vi "Arm State Machine.vi"   [LabVIEW 2015]
uses:
  ArmStates.ctl
  <vilib>/Rock Robotics/WPI/DriverStation/WPI_DriverStationRobotMode2.ctl
  Robot Global Data.vi
  <vilib>/Rock Robotics/WPI/Utilities/WPI_GetSetVariantRefNum.vi
types:
  T1 = typedef "ArmStates.ctl" = enum16{"Arm Drive Position", "Winch Up", "Level Arm", "Hold Climb", "Drawbridge Drive Forward", "Shoot Position", "Roll Out", "Hic Up Rollers Off", "Draw Bridge Arm Down", "Harvest Back Down", "Harvest Hic up", "Portcullis", "Sally Door", "Harvest", "Arm Up", "Arm Down"}
  T2 = cluster{"Arm State":T1, "Current Arm Position":dbl, "Arm Base Offset":dbl, "Arm Up Position":dbl, "Sally Door Position":dbl, "Porticullis Position":dbl, "Drawbridge Position":dbl, "Drive Position":dbl, "Arm Hic Up Position":dbl, "Desired Arm Position":dbl, "Arm Power Vbus":bool, "Roller":bool, "Hic Up Counter":i32, "Right Drive Overide Speed":dbl, "Left Drive Overide Speed":dbl, "Overide Drives":bool, "Roller Speed":dbl, "PTO on":bool, "PTO break Off":bool, "Current Encoder Position":dbl, "Starting Encoder Position":dbl, "Last State":T1, "Arm Hold Cylinder":bool, "New Base Offset":bool}
  T3 = typedef "WPI_MotorControlDeviceRef.ctl" = cluster{"DeviceStatus":errorcluster, "Type":T4, "PWM":cluster{"PWM Channel":T5, "DeadBand":T6}, "CAN":cluster{"Device Number":u8, "Control Mode":T7, "Semaphore":T8, "Max Vout":dbl, "TalonSRX Control Mode":T9}, "Invert":bool}
  T4 = typedef "WPI_MotorControlType.ctl" = enum16{"PWM", "CAN", "CANTalonSRX"}
  T5 = typedef "FPGA_DIOPWMChannel.ctl" = enum8{"PWM 0", "PWM 1", "PWM 2", "PWM 3", "PWM 4", "PWM 5", "PWM 6", "PWM 7", "PWM 8", "PWM 9", "PWM MXP 0", "PWM MXP 1", "PWM MXP 2", "PWM MXP 3", "PWM MXP 4", "PWM MXP 5", "PWM MXP 6", "PWM MXP 7", "PWM MXP 8", "PWM MXP 9", "Invalid"}
  T6 = typedef "WPI_PWMDeadband.ctl" = cluster{"Name":string, "maxPositivePwm":i32, "minPositivePwm":i32, "centerPwm":i32, "maxNegativePwm":i32, "minNegativePwm":i32, "angularRange":u16}
  T7 = typedef "WPI_CANJaguar_ControlMode.ctl" = enum8{"Percent VBus", "Current", "Speed", "Position", "Voltage"}
  T8 = typedef "Semaphore RefNum" = refnum<k1>
  T9 = typedef "WPI_CANTalonSRX_APIControlMode.ctl" = enum8{"Percent VBus", "Speed", "Position", "Slave", "Unchanged / Invalid", "Voltage Compensation", "Current", "Motion Profile"}
  T10 = typedef "WPI_CANTalonSRX_GlobalStatus.ctl" = cluster{"Applied Throttle":dbl, "Module Enabled":bool, "CAN Error":errorcluster, "Closed Loop Error":dbl, "Forward Limit Switch Closed":bool, "Reverse Limit Switch Closed":bool, "Sensor Position":dbl, "Sensor Velocity":dbl, "Current":dbl, "Sticky Fault - Over Temp":bool, "Sticky Fault - Under Voltage":bool, "Sticky Fault - Forward Limit":bool, "Sticky Fault - Reverse Limit":bool, "Sticky Fault - Forward Soft Limit":bool, "Sticky Fault - Reverse Soft Limit":bool, "Brake is Enabled":bool, "Encoder Position":dbl, "Encoder Velocity":dbl, "Encoder Index Count":dbl, "Encoder A Pin State":bool, "Encoder B Pin State":bool, "Encoder Index Pin State":bool, "Analog In":dbl, "Analog In Velocity":dbl, "Temperature (C)":dbl, "Battery Voltage":dbl, "Control 5 Is Supported":bool, "Current Profile Slot Select":dbl, "Pos Div 8":bool, "Vel Div 4":bool, "Pulse Width Position":i32, "Pulse Width Velocity":i32, "Pulse Width Rise To Rise (us)":i32, "Pulse Width Rise To Fall (us)":i32, "Mot Prof Active Is Under Run":bool, "Mot Prof Active Has Under Run":bool, "Mot Prof Active Is Last":bool, "Mot Prof Active Velocity Only":bool, "Mot Prof Active Is Valid":bool, "Mot Prof Buffer Is Full":bool, "Mot Prof Active Profile Slot Select":i32, "Mot Prof NextID":i32, "Mot Prof Count":i32, "Mot Prof Active Velocity":dbl, "Mot Prof Active Position":dbl, "Mot Prof Output Enable":i32}
  T11 = typedef "WPI_DriverStationRobotMode2.ctl" = enum16{"Autonomous Disabled", "Autonomous Enabled", "Teleop Disabled", "Teleop Enabled", "Disconnected", "Finish", "Test Disabled", "Test Enabled", "Emergency Stopped"}
  T12 = typedef "WPI_JoystickDevRef.ctl" = cluster{"Device":T13}
  T13 = typedef "WPI_JoystickDeviceEnum.ctl" = enum16{"USB 0", "USB 1", "USB 2", "USB 3", "USB 4", "USB 5"}
  T14 = cluster{"Buttons[0]":bool, "Buttons[1]":bool, "Buttons[2]":bool, "Buttons[3]":bool, "Buttons[4]":bool, "Buttons[5]":bool, "Buttons[6]":bool, "Buttons[7]":bool, "Buttons[8]":bool}
  T15 = typedef "WPI_SwitchDevRef.ctl" = cluster{"DevStatus":errorcluster, "DIO Channel":T16, "CntIndex":T17, "Normally Closed":bool}
  T16 = typedef "FPGA_DIOChannel.ctl" = enum8{"DIO 0", "DIO 1", "DIO 2", "DIO 3", "DIO 4", "DIO 5", "DIO 6", "DIO 7", "DIO 8", "DIO 9", "DIO MXP 0", "DIO MXP 1", "DIO MXP 2", "DIO MXP 3", "DIO MXP 4", "DIO MXP 5", "DIO MXP 6", "DIO MXP 7", "DIO MXP 8", "DIO MXP 9", "DIO MXP 10", "DIO MXP 11", "DIO MXP 12", "DIO MXP 13", "DIO MXP 14", "DIO MXP 15", "Invalid"}
  T17 = typedef "FPGA_CounterCtrSystemIndex.ctl" = enum8{"Ctr 0", "Ctr 1", "Ctr 2", "Ctr 3", "Ctr 4", "Ctr 5", "Ctr 6", "Ctr 7", "Invalid"}
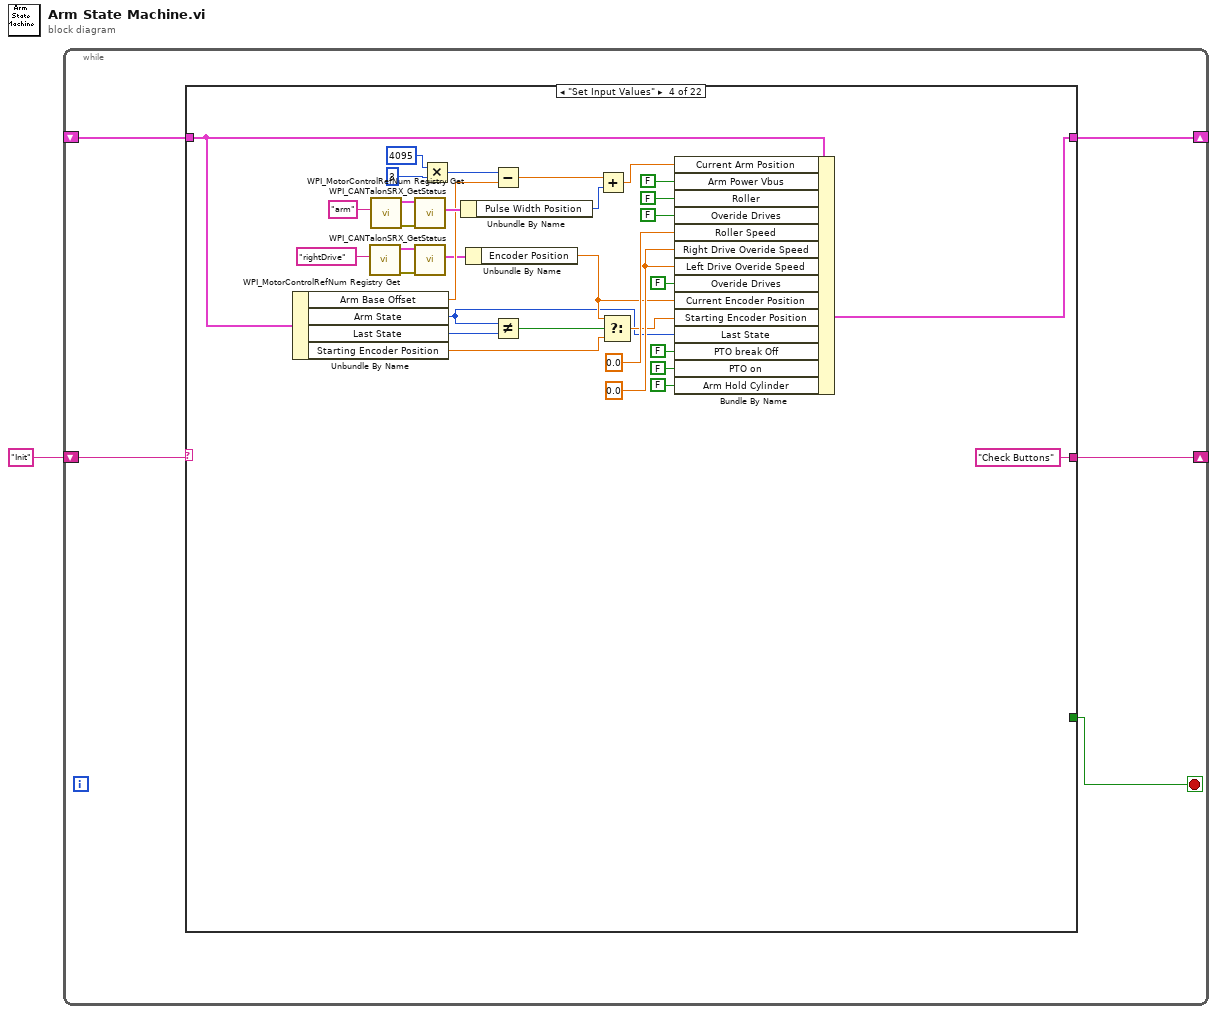
[diagram p0: block diagram]
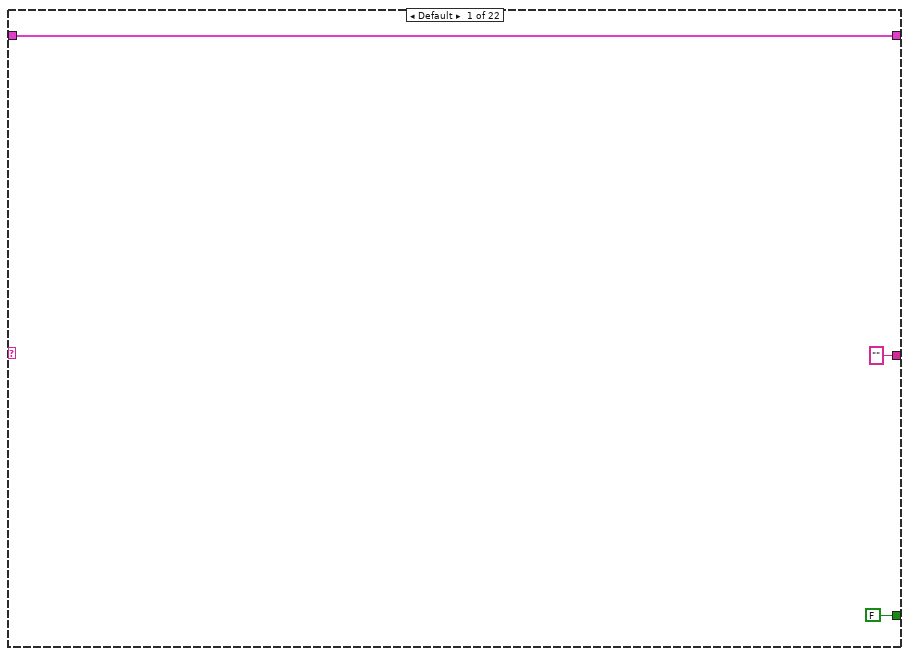
[diagram p2: hidden frame]
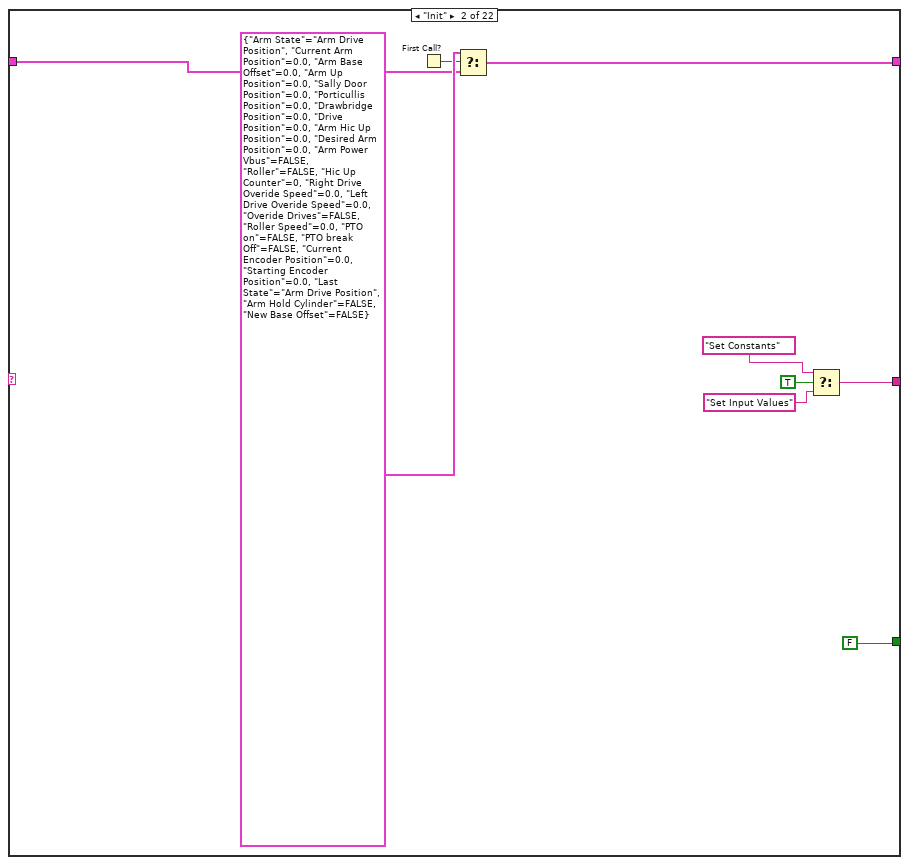
[diagram p3: hidden frame]
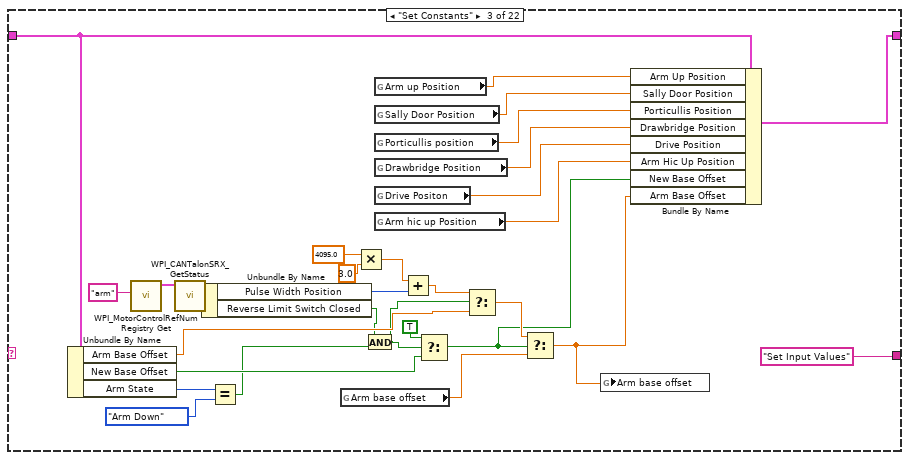
[diagram p4: hidden frame]
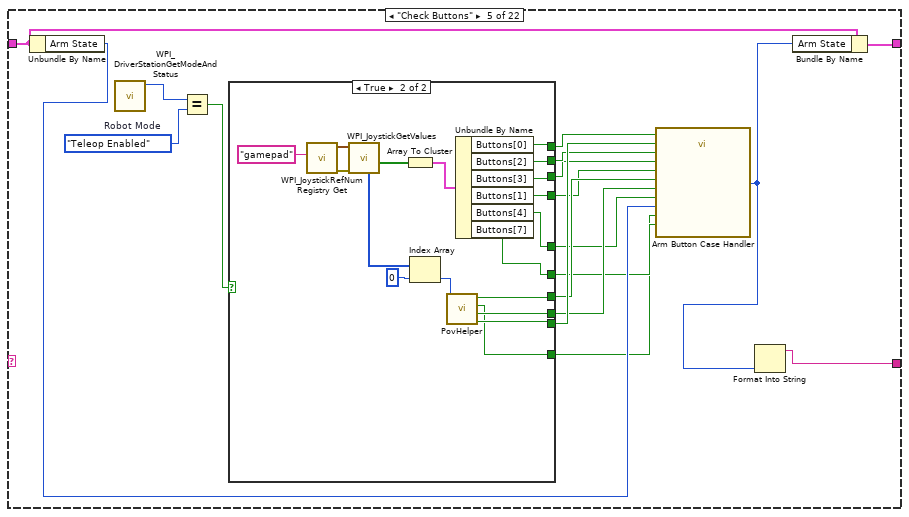
[diagram p5: hidden frame]
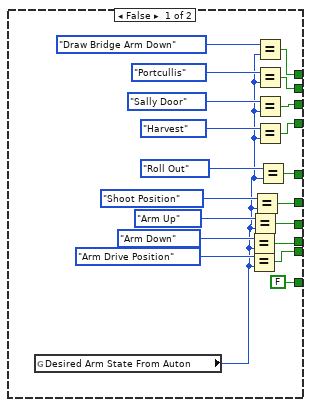
[diagram p6: hidden frame]
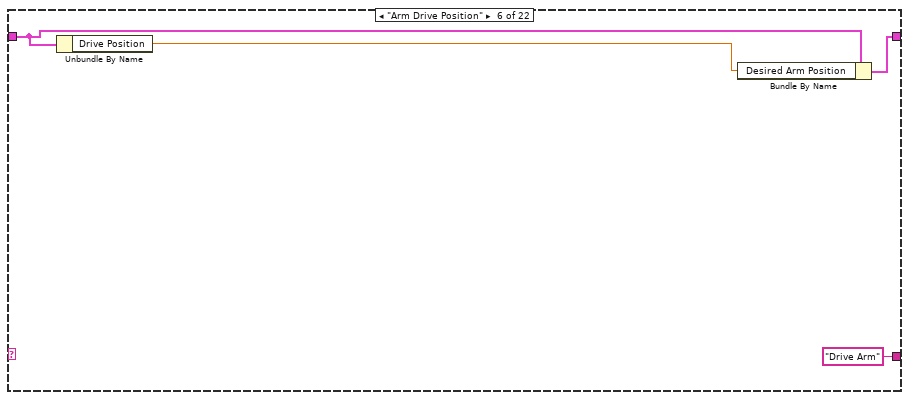
[diagram p7: hidden frame]
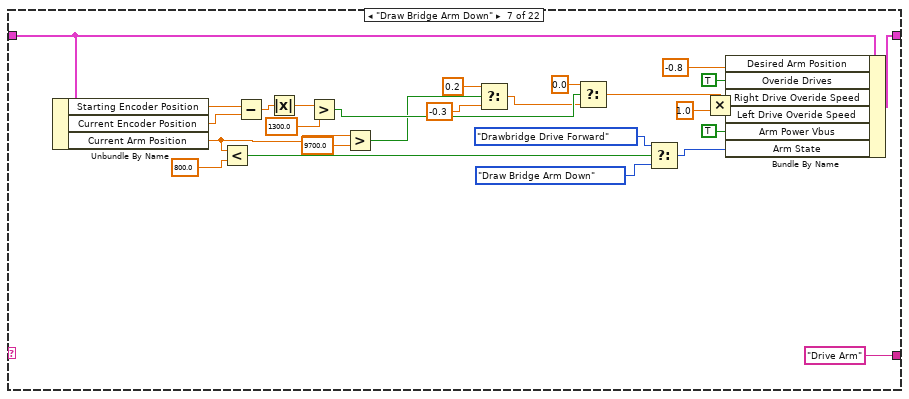
[diagram p8: hidden frame]
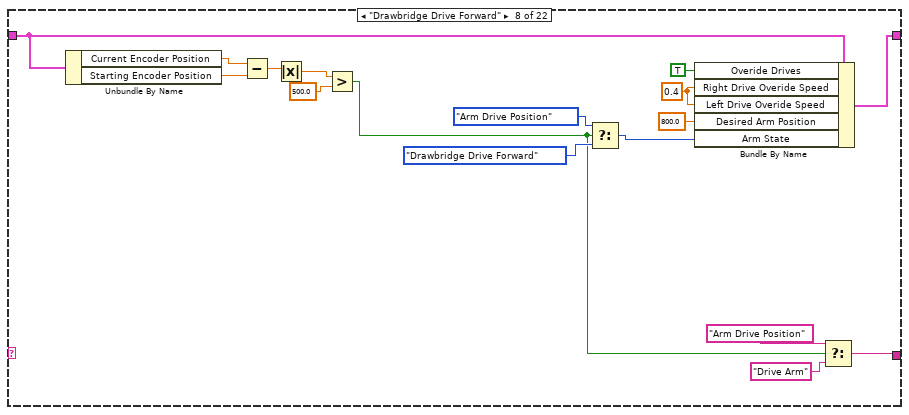
[diagram p9: hidden frame]
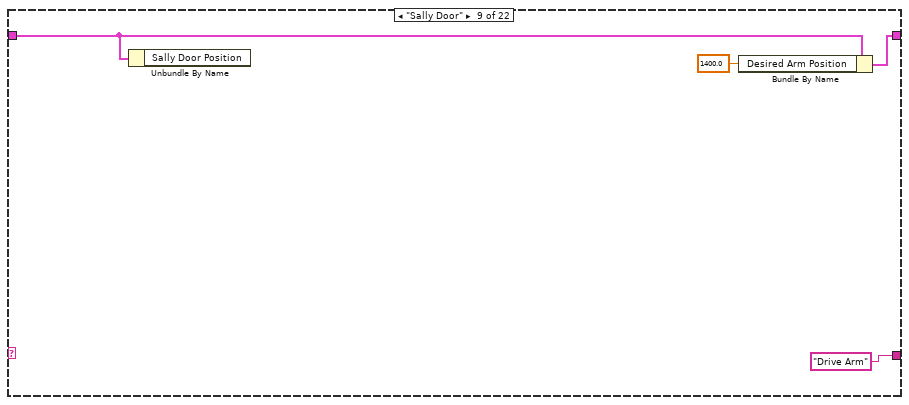
[diagram p10: hidden frame]
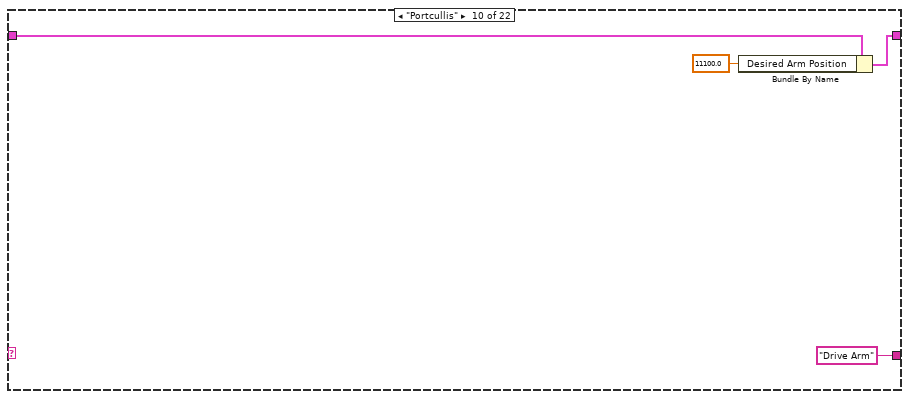
[diagram p11: hidden frame]
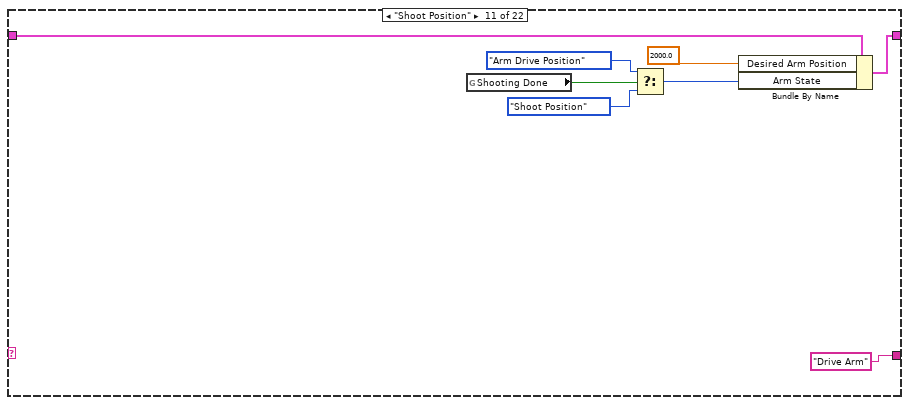
[diagram p12: hidden frame]
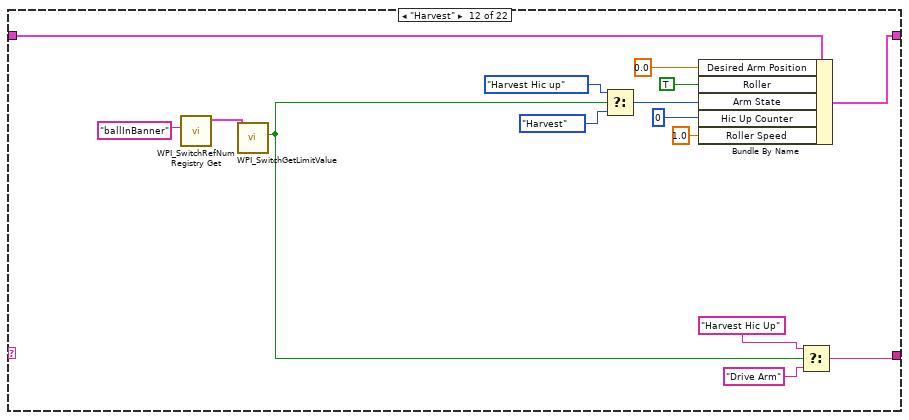
[diagram p13: hidden frame]
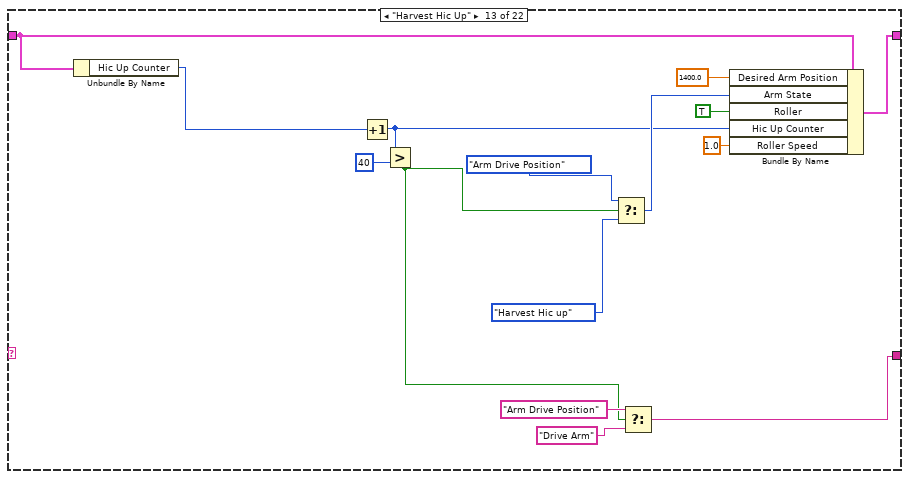
[diagram p14: hidden frame]
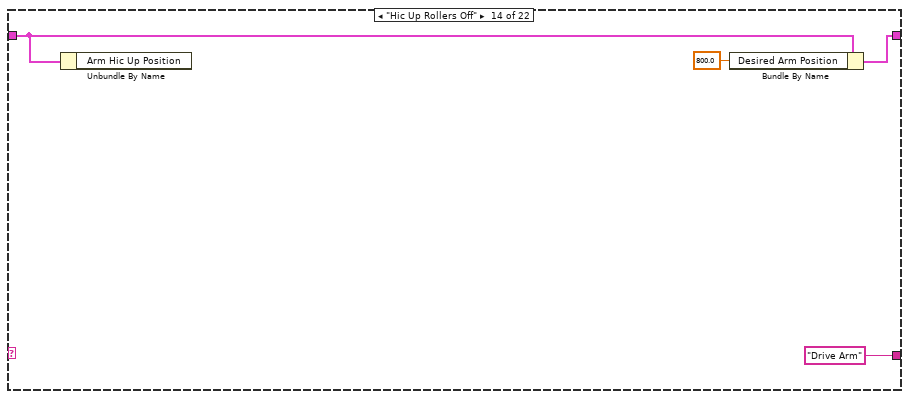
[diagram p15: hidden frame]
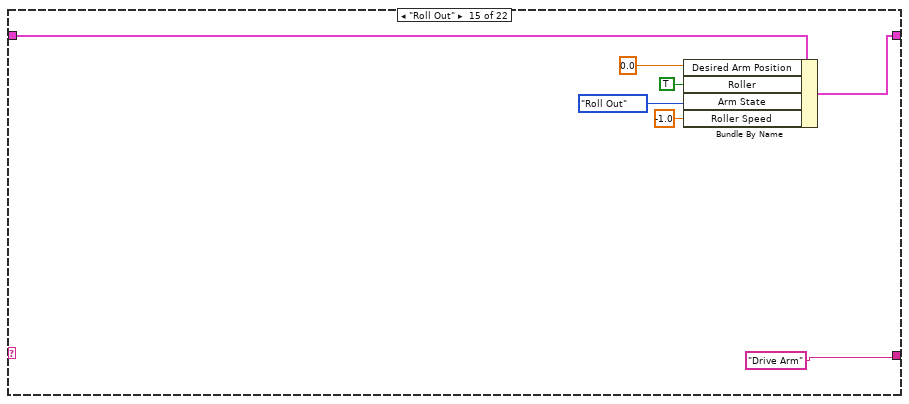
[diagram p16: hidden frame]
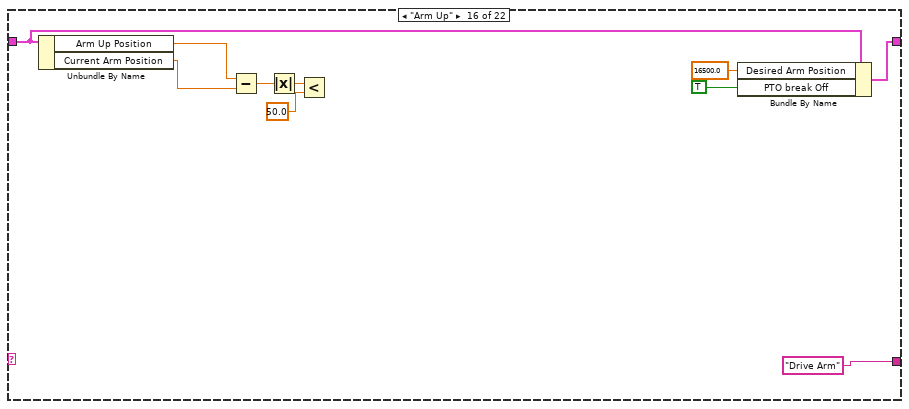
[diagram p17: hidden frame]
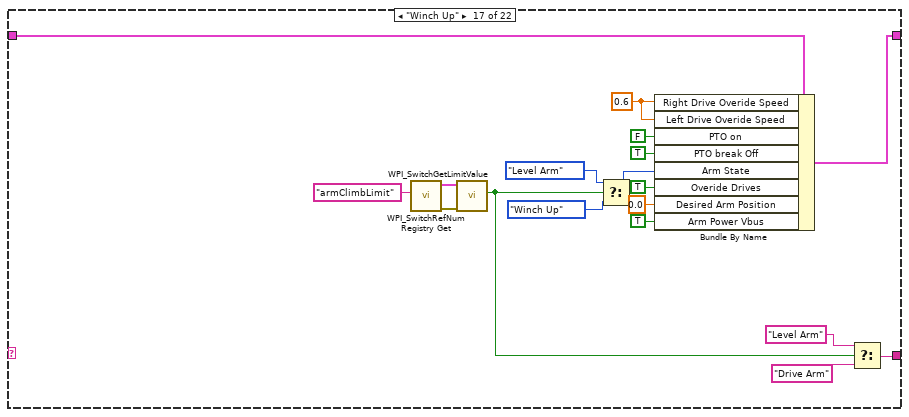
[diagram p18: hidden frame]
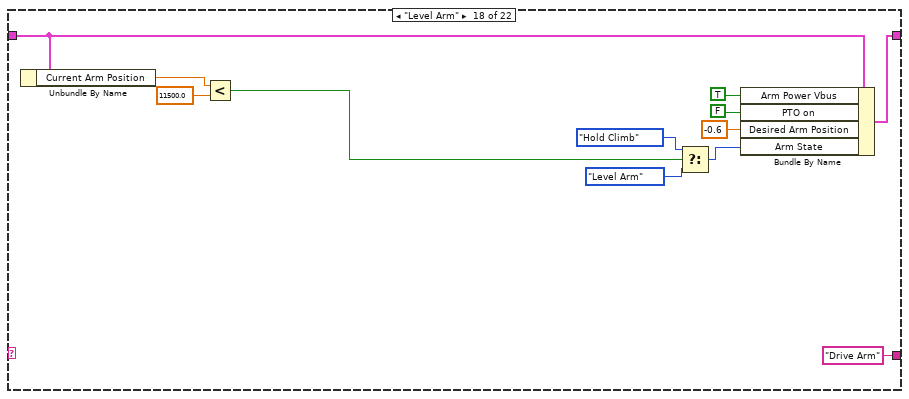
[diagram p19: hidden frame]
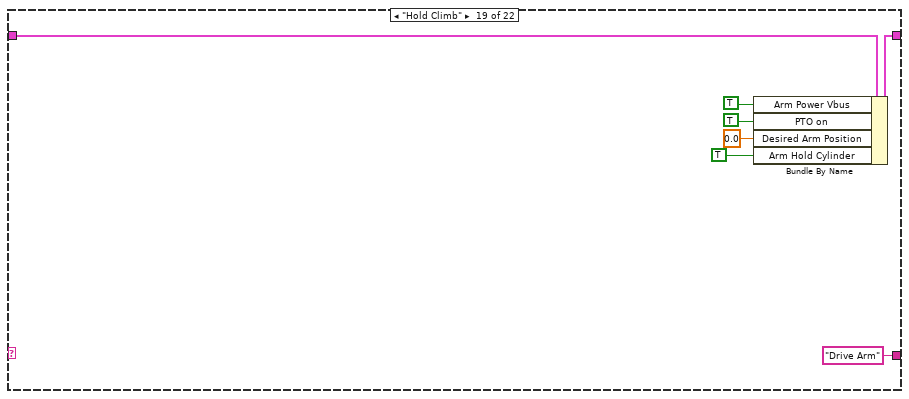
[diagram p20: hidden frame]
diagram:
  n1 = while {
    shift-right: [w3] -> _
    shift-left: "Init" -> [w6]
    shift-right: [w5] -> _
    shift-left: _ -> [w4]
    stop <- w2 stop-if-true
    n2 = case shown="\"Set Input Values\"" w6 {
      tunnel: [w8 w17 w46 w80 w90 w139 w167 w183 w187 w191 w199 w209 w229 w233 w240 w250 w268 w280 w284 w291 w306 w307] -> w5
      tunnel: w4 -> [w8 w16 w39 w72 w91 w140 w164 w184 w186 w190 w198 w210 w230 w234 w241 w251 w269 w281 w285 w292 w306 w307]
      tunnel: ["" w15 "Set Input Values" "Check Buttons" w82 "Drive Arm" "Drive Arm" w169 "Drive Arm" "Drive Arm" "Drive Arm" w211 w223 "Drive Arm" "Drive Arm" "Drive Arm" w258 "Drive Arm" ("t") "Drive Arm" ("t") "Drive Arm" "Exit" _] -> w3
      tunnel: [FALSE FALSE _ _ _ _ _ _ _ _ _ _ _ _ _ _ _ _ _ _ TRUE TRUE] -> w2
      frame Default {
      }
      frame "Init" {
        n3 = First Call?() -> (First Call?: T/F=w12:bool)
        n4 = Select(t=T2 {"Arm State"=enum."Arm Drive Position", "Current Arm Position"=0.0, "Arm Base Offset"=0.0, "Arm Up Position"=0.0, "Sally Door Position"=0.0, "Porticullis Position"=0.0, "Drawbridge Position"=0.0, "Drive Position"=0.0, "Arm Hic Up Position"=0.0, "Desired Arm Position"=0.0, "Arm Power Vbus"=FALSE, "Roller"=FALSE, "Hic Up Counter"=0, "Right Drive Overide Speed"=0.0, "Left Drive Overide Speed"=0.0, "Overide Drives"=FALSE, "Roller Speed"=0.0, "PTO on"=FALSE, "PTO break Off"=FALSE, "Current Encoder Position"=0.0, "Starting Encoder Position"=0.0, "Last State"=enum."Arm Drive Position", "Arm Hold Cylinder"=FALSE, "New Base Offset"=FALSE}, s=w12, f=w16) -> (s? t:f=w17:T2)
        n5 = Select(t="Set Constants", s=TRUE, f="Set Input Values") -> (s? t:f=w15:string)
      }
      frame "Set Constants" {
        n6 = Unbundle By Name(w39) -> ("Arm Base Offset"=w27:dbl, "New Base Offset"=w38:bool, "Arm State"=w23:T1)
        n7 = call <vilib>:"WPI_MotorControlRefNum Registry Get.vi"("refnum name"="arm") -> ("MotorControlDevRef"=w32:T3)  [unwired: 9 in, 1 out]
        n8 = call <vilib>:"WPI_CANTalonSRX_GetStatus.vi"("CAN Talon SRX Ref"=w32) -> ("Talon SRX Status"=w30:T10)  [unwired: 8 in, 2 out]
        n9 = Unbundle By Name(w30) -> ("Pulse Width Position"=w31:i32, "Reverse Limit Switch Closed"=w19:bool)
        n10 = Equal?(x=w23, y=ArmStates."Arm Down" ("Arm State")) -> (x = y?=w21:bool)
        n11 = global read "Robot Global Data.vi" "Arm base offset"() -> (w36:dbl)
        n12 = Multiply(x=4095.0, y=3.0) -> (x*y=w33:dbl)
        n13 = And(x=w19, y=w21) -> (x .and. y?=w20:bool)
        n14 = global read "Robot Global Data.vi" "Arm up Position"() -> (w45:dbl)
        n15 = global read "Robot Global Data.vi" "Sally Door Position"() -> (w44:dbl)
        n16 = global read "Robot Global Data.vi" "Porticullis position"() -> (w43:dbl)
        n17 = global read "Robot Global Data.vi" "Drawbridge Position"() -> (w42:dbl)
        n18 = global read "Robot Global Data.vi" "Drive Positon"() -> (w40:dbl)
        n19 = global read "Robot Global Data.vi" "Arm hic up Position"() -> (w41:dbl)
        n20 = Add(x=w33, y=w31) -> (x+y=w28:dbl)
        n21 = Select(t=TRUE, s=w20, f=w38) -> (s? t:f=w25:bool)
        n22 = Select(t=w28, s=w20, f=w27) -> (s? t:f=w26:dbl)
        n23 = Select(t=w26, s=w25, f=w36) -> (s? t:f=w24:dbl)
        n24 = global write "Robot Global Data.vi" "Arm base offset"(w24) -> ()
        n25 = Bundle By Name(cluster=w39, "Arm Up Position"=w45, "Sally Door Position"=w44, "Porticullis Position"=w43, "Drawbridge Position"=w42, "Drive Position"=w40, "Arm Hic Up Position"=w41, "New Base Offset"=w25, "Arm Base Offset"=w24) -> (w46:T2)
      }
      frame "Set Input Values" {
        w62 = 0.0 ("Roller Speed")
        n26 = Unbundle By Name(w72) -> ("Arm Base Offset"=w71:dbl, "Arm State"=w51:T1, "Last State"=w56:T1, "Starting Encoder Position"=w54:dbl)
        n27 = call <vilib>:"WPI_MotorControlRefNum Registry Get.vi"("refnum name"="rightDrive") -> ("error out"=w60:errorcluster, "MotorControlDevRef"=w59:T3)  [unwired: 9 in]
        n28 = call <vilib>:"WPI_MotorControlRefNum Registry Get.vi"("refnum name"="arm") -> ("error out"=w78:errorcluster, "MotorControlDevRef"=w79:T3)  [unwired: 9 in]
        n29 = call <vilib>:"WPI_CANTalonSRX_GetStatus.vi"("error in (no error)"=w78, "CAN Talon SRX Ref"=w79) -> ("Talon SRX Status"=w76:T10)  [unwired: 7 in, 2 out]
        n30 = call <vilib>:"WPI_CANTalonSRX_GetStatus.vi"("error in (no error)"=w60, "CAN Talon SRX Ref"=w59) -> ("Talon SRX Status"=w58:T10)  [unwired: 7 in, 2 out]
        n31 = Multiply(x=4095, y=3) -> (x*y=w73:i32)
        n32 = Unbundle By Name(w76) -> ("Pulse Width Position"=w69:i32)
        n33 = Unbundle By Name(w58) -> ("Encoder Position"=w53:dbl)
        n34 = Subtract(x=w73, y=w71) -> (x-y=w70:dbl)
        n35 = Not Equal?(x=w51, y=w56) -> (x != y?=w55:bool)
        n36 = Add(x=w70, y=w69) -> (x+y=w68:dbl)
        n37 = Select(t=w53, s=w55, f=w54) -> (s? t:f=w52:dbl)
        n38 = Bundle By Name(cluster=w72, "Current Arm Position"=w68, "Arm Power Vbus"=FALSE, "Roller"=FALSE, "Overide Drives"=FALSE, "Roller Speed"=0.0, "Right Drive Overide Speed"=w62, "Left Drive Overide Speed"=w62, "Overide Drives"=FALSE, "Current Encoder Position"=w53, "Starting Encoder Position"=w52, "Last State"=w51, "PTO break Off"=FALSE ("PTO break on"), "PTO on"=FALSE, "Arm Hold Cylinder"=FALSE) -> (w80:T2)
      }
      frame "Check Buttons" {
        w97 = WPI_DriverStationRobotMode2."Teleop Enabled"  # Robot Mode
        n39 = Unbundle By Name(w91) -> ("Arm State"=w86:T1)
        n40 = call <vilib>:"WPI_DriverStationGetModeAndStatus.vi"() -> ("Robot Mode"=w98:T11)  [unwired: 10 in, 1 out]
        n41 = Equal?(x=w98, y=w97) -> (x = y?=w96:bool)
        n42 = case shown="True" w96 {
          tunnel: [w118 w120] -> w95
          tunnel: [w102 w126] -> w94
          tunnel: [w115 w128] -> w88
          tunnel: [w100 w127] -> w87
          tunnel: [w116 w125] -> w89
          tunnel: [w104 w124] -> w93
          tunnel: [w103 w123] -> w92
          tunnel: [w106 w122] -> w85
          tunnel: [w105 w121] -> w84
          tunnel: [FALSE ("Right arrow") w119] -> w81
          frame False {
            n43 = global read "Robot Global Data.vi" "Desired Arm State From Auton"() -> (w101:T1)
            n44 = Equal?(x=ArmStates."Arm Down" ("Arm State"), y=w101) -> (x = y?=w103:bool)
            n45 = Equal?(x=ArmStates."Arm Drive Position" ("Arm State"), y=w101) -> (x = y?=w102:bool)
            n46 = Equal?(x=ArmStates."Arm Up" ("Arm State"), y=w101) -> (x = y?=w104:bool)
            n47 = Equal?(x=ArmStates."Shoot Position" ("Arm State"), y=w101) -> (x = y?=w105:bool)
            n48 = Equal?(x=ArmStates."Draw Bridge Arm Down" ("Arm State"), y=w101) -> (x = y?=w118:bool)
            n49 = Equal?(x=ArmStates."Portcullis" ("Arm State"), y=w101) -> (x = y?=w116:bool)
            n50 = Equal?(x=ArmStates."Sally Door" ("Arm State"), y=w101) -> (x = y?=w115:bool)
            n51 = Equal?(x=ArmStates."Harvest" ("Arm State"), y=w101) -> (x = y?=w100:bool)
            n52 = Equal?(x=ArmStates."Roll Out" ("Arm State"), y=w101) -> (x = y?=w106:bool)
          }
          frame True {
            n53 = call <vilib>:"WPI_JoystickRefNum Registry Get.vi"("refnum name"="gamepad") -> ("error out"=w136:errorcluster, "JoystickDevRef"=w135:T12)  [unwired: 9 in]
            n54 = call <vilib>:"WPI_JoystickGetValues.vi"("error in (no error)"=w136, "JoystickDevRef"=w135) -> ("Buttons"=w132:bool[], "POVs"=w131:i16[])  [unwired: 5 in, 3 out]
            n55 = Array To Cluster(array=w132) -> (cluster=w133:T14)
            n56 = Index Array(array=w131, index=0) -> (element=w129:i16)
            n57 = call "PovHelper.vi"("Input POV"=w129) -> ("Left arrow"=w126:bool, "Down arrow"=w123:bool, "Right arrow"=w119:bool, "Top arrow"=w124:bool)  [unwired: 7 in]
            n58 = Unbundle By Name(w133) -> ("Buttons[0]"=w120:bool, "Buttons[2]"=w125:bool, "Buttons[3]"=w128:bool, "Buttons[1]"=w127:bool, "Buttons[4]"=w122:bool, "Buttons[7]"=w121:bool)
          }
        }
        n59 = call "Arm Button Case Handler.vi"("Draw Bridge"=w95, "Arm Drive Position"=w94, "Portcullis"=w89, "Sally Door"=w88, "Harvest"=w87, "Arm Up"=w93, "Shoot Position"=w84, "Arm Down"=w92, "Roll Out"=w85, "Current Arm State"=w86, "Winch Up"=w81) -> ("Arm state"=w83:T1)  [unwired: 8 in]
        n60 = Format Into String(w83) -> (resulting string=w82:string)  [unwired: 3 in, 1 out]
        n61 = Bundle By Name(cluster=w91, "Arm State"=w83) -> (w90:T2)
      }
      frame "Arm Drive Position" {
        n62 = Unbundle By Name(w140) -> ("Drive Position"=w138:dbl)
        n63 = Bundle By Name(cluster=w140, "Desired Arm Position"=w138) -> (w139:T2)
      }
      frame "Draw Bridge Arm Down" {
        n64 = Unbundle By Name(w164) -> ("Starting Encoder Position"=w159:dbl, "Current Encoder Position"=w158:dbl, "Current Arm Position"=w151:dbl)
        n65 = Less?(x=w151, y=800.0 ("Current Arm Position")) -> (x < y?=w160:bool)
        n66 = Subtract(x=w159, y=w158) -> (x-y=w157:dbl)
        n67 = Absolute Value(x=w157) -> (abs(x)=w156:dbl)
        n68 = Greater?(x=w156, y=1300.0) -> (0:w148:bool)
        n69 = Greater?(x=w151, y=9700.0) -> (0:w146:bool)
        n70 = Select(t=0.2, s=w146, f=-0.3 ("Drawbridge Drive Power")) -> (s? t:f=w147:dbl)
        n71 = Select(t=0.0, s=w148, f=w147) -> (s? t:f=w153:dbl)
        n72 = Select(t=ArmStates."Drawbridge Drive Forward" ("Arm State"), s=w160, f=ArmStates."Draw Bridge Arm Down" ("Arm State")) -> (s? t:f=w163:T1)
        n73 = Multiply(x=w153, y=1.0) -> (x*y=w142:dbl)
        n74 = Bundle By Name(cluster=w164, "Desired Arm Position"=-0.8 ("Arm Drive Speed"), "Overide Drives"=TRUE, "Right Drive Overide Speed"=w153, "Left Drive Overide Speed"=w142, "Arm Power Vbus"=TRUE, "Arm State"=w163) -> (w167:T2)
      }
      frame "Drawbridge Drive Forward" {
        w181 = 0.4 ("Right Drive Overide Speed")
        n75 = Unbundle By Name(w184) -> ("Current Encoder Position"=w178:dbl, "Starting Encoder Position"=w179:dbl)
        n76 = Subtract(x=w178, y=w179) -> (x-y=w177:dbl)
        n77 = Absolute Value(x=w177) -> (abs(x)=w176:dbl)
        n78 = Greater?(x=w176, y=500.0) -> (0:w168:bool)
        n79 = Select(t=ArmStates."Arm Drive Position" ("Arm State"), s=w168, f=ArmStates."Drawbridge Drive Forward" ("Arm State")) -> (s? t:f=w172:T1)
        n80 = Bundle By Name(cluster=w184, "Overide Drives"=TRUE, "Right Drive Overide Speed"=w181, "Left Drive Overide Speed"=w181, "Desired Arm Position"=800.0, "Arm State"=w172) -> (w183:T2)
        n81 = Select(t="Arm Drive Position", s=w168, f="Drive Arm") -> (s? t:f=w169:string)
      }
      frame "Sally Door" {
        n82 = Unbundle By Name(w186) -> ()  [unwired: 1 out]
        n83 = Bundle By Name(cluster=w186, "Desired Arm Position"=1400.0) -> (w187:T2)
      }
      frame "Portcullis" {
        n84 = Bundle By Name(cluster=w190, "Desired Arm Position"=11100.0) -> (w191:T2)
      }
      frame "Shoot Position" {
        n85 = global read "Robot Global Data.vi" "Shooting Done"() -> (w194:bool)
        n86 = Select(t=ArmStates."Arm Drive Position" ("Arm State"), s=w194, f=ArmStates."Shoot Position" ("Arm State")) -> (s? t:f=w193:T1)
        n87 = Bundle By Name(cluster=w198, "Desired Arm Position"=2000.0, "Arm State"=w193) -> (w199:T2)
      }
      frame "Harvest" {
        n88 = call <vilib>:"WPI_SwitchRefNum Registry Get.vi"("refnum name"="ballInBanner") -> ("SwitchDevRef"=w205:T15)  [unwired: 9 in, 1 out]
        n89 = call <vilib>:"WPI_SwitchGetLimitValue.vi"("SwitchDevRef"=w205) -> ("Switch Pressed"=w203:bool)  [unwired: 8 in, 2 out]
        n90 = Select(t=ArmStates."Harvest Hic up" ("Arm State"), s=w203, f=ArmStates."Harvest" ("Arm State")) -> (s? t:f=w208:T1)
        n91 = Bundle By Name(cluster=w210, "Desired Arm Position"=0.0, "Roller"=TRUE, "Arm State"=w208, "Hic Up Counter"=0, "Roller Speed"=1.0) -> (w209:T2)
        n92 = Select(t="Harvest Hic Up", s=w203, f="Drive Arm") -> (s? t:f=w211:string)
      }
      frame "Harvest Hic Up" {
        n93 = Unbundle By Name(w230) -> ("Hic Up Counter"=w221:i32)
        n94 = Increment(x=w221) -> (x+1=w220:i32)
        n95 = Greater?(x=w220, y=40) -> (0:w218:bool)
        n96 = Select(t=ArmStates."Arm Drive Position" ("Arm State"), s=w218, f=ArmStates."Harvest Hic up" ("Arm State")) -> (s? t:f=w222:T1)
        n97 = Select(t="Arm Drive Position", s=w218, f="Drive Arm") -> (s? t:f=w223:string)
        n98 = Bundle By Name(cluster=w230, "Desired Arm Position"=1400.0, "Arm State"=w222, "Roller"=TRUE ("Arm Power Vbus"), "Hic Up Counter"=w220, "Roller Speed"=1.0) -> (w229:T2)
      }
      frame "Hic Up Rollers Off" {
        n99 = Unbundle By Name(w234) -> ()  [unwired: 1 out]
        n100 = Bundle By Name(cluster=w234, "Desired Arm Position"=800.0) -> (w233:T2)
      }
      frame "Roll Out" {
        n101 = Bundle By Name(cluster=w241, "Desired Arm Position"=0.0, "Roller"=TRUE, "Arm State"=ArmStates."Roll Out", "Roller Speed"=-1.0) -> (w240:T2)
      }
      frame "Arm Up" {
        n102 = Unbundle By Name(w251) -> ("Arm Up Position"=w247:dbl, "Current Arm Position"=w246:dbl)
        n103 = Subtract(x=w247, y=w246) -> (x-y=w245:dbl)
        n104 = Absolute Value(x=w245) -> (abs(x)=w244:dbl)
        n105 = Less?(x=w244, y=50.0) -> ()  [unwired: 1 out]
        n106 = Bundle By Name(cluster=w251, "Desired Arm Position"=16500.0, "PTO break Off"=TRUE ("PTO break on")) -> (w250:T2)
      }
      frame "Winch Up" {
        w265 = 0.6 ("Right Drive Overide Speed")
        n107 = call <vilib>:"WPI_SwitchRefNum Registry Get.vi"("refnum name"="armClimbLimit") -> ("error out"=w261:errorcluster, "SwitchDevRef"=w260:T15)  [unwired: 9 in]
        n108 = call <vilib>:"WPI_SwitchGetLimitValue.vi"("error in (no error)"=w261, "SwitchDevRef"=w260) -> ("Switch Pressed"=w255:bool)  [unwired: 7 in, 2 out]
        n109 = Select(t=ArmStates."Level Arm" ("Arm State"), s=w255, f=ArmStates."Winch Up" ("Arm State")) -> (s? t:f=w264:T1)
        n110 = Bundle By Name(cluster=w269, "Right Drive Overide Speed"=w265, "Left Drive Overide Speed"=w265, "PTO on"=FALSE, "PTO break Off"=TRUE ("PTO break on"), "Arm State"=w264, "Overide Drives"=TRUE, "Desired Arm Position"=0.0, "Arm Power Vbus"=TRUE) -> (w268:T2)
        n111 = Select(t="Level Arm", s=w255, f="Drive Arm") -> (s? t:f=w258:string)
      }
      frame "Level Arm" {
        n112 = Unbundle By Name(w281) -> ("Current Arm Position"=w276:dbl)
        n113 = Less?(x=w276, y=11500.0) -> (x < y?=w271:bool)
        n114 = Select(t=ArmStates."Hold Climb" ("Arm State"), s=w271, f=ArmStates."Level Arm" ("Arm State")) -> (s? t:f=w272:T1)
        n115 = Bundle By Name(cluster=w281, "Arm Power Vbus"=TRUE, "PTO on"=FALSE, "Desired Arm Position"=-0.6, "Arm State"=w272) -> (w280:T2)
      }
      frame "Hold Climb" {
        n116 = Bundle By Name(cluster=w285, "Arm Power Vbus"=TRUE, "PTO on"=TRUE, "Desired Arm Position"=0.0, "Arm Hold Cylinder"=TRUE) -> (w284:T2)
      }
      frame "Arm Down" {
        n117 = Bundle By Name(cluster=w292, "Desired Arm Position"=0.0) -> (w291:T2)
      }
      frame "Drive Arm" {
        n118 = Unbundle By Name(w306) -> ("Desired Arm Position"=w305:dbl, "Arm Power Vbus"=w304:bool, "Roller"=w303:bool, "Arm State"=w300:T1, "Roller Speed"=w299:dbl, "Overide Drives"=w298:bool, "Right Drive Overide Speed"=w297:dbl, "Left Drive Overide Speed"=w296:dbl, "PTO on"=w295:bool, "PTO break Off"=w294:bool, "Arm Hold Cylinder"=w293:bool)
        n119 = global write "Robot Global Data.vi" "Desired Arm Position"(w305) -> ()
        n120 = global write "Robot Global Data.vi" "Arm Power Vbus"(w304) -> ()
        n121 = global write "Robot Global Data.vi" "Roller"(w303) -> ()
        n122 = global write "Robot Global Data.vi" "Arm State"(w300) -> ()
        n123 = global write "Robot Global Data.vi" "Roller speed"(w299) -> ()
        n124 = global write "Robot Global Data.vi" "Overide Drives"(w298) -> ()
        n125 = global write "Robot Global Data.vi" "Right Drive Overide"(w297) -> ()
        n126 = global write "Robot Global Data.vi" "Left Drive Overide"(w296) -> ()
        n127 = global write "Robot Global Data.vi" "Pto on"(w295) -> ()
        n128 = global write "Robot Global Data.vi" "Pto break on"(w294) -> ()
        n129 = global write "Robot Global Data.vi" "Arm Hold Cylinder"(w293) -> ()
      }
      frame "Exit" {
      }
    }
  }
